vi "InitFittedCurvePolynom.vi"   [LabVIEW 2013]
uses:
  GlobalVariables/FittedCurvePolynom.vi
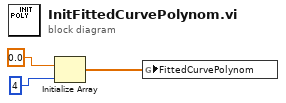
[diagram p0: block diagram]
diagram:
  n1 = Initialize Array(0.0, 4) -> (w1:dbl[])
  n2 = global write "FittedCurvePolynom.vi" "FittedCurvePolynom"(w1) -> ()
